vi "MdfCreateDataGroup.vi"(8 "error in (no error)":errorcluster, 10 "ChannelGroupName":string="MDFCGName", 11 "MDFRef":refnum<k24>) -> (0 "error IO":errorcluster, 2 "ChannelGroup":refnum<k24>, 3 "MDFRef out":refnum<k24>)   [LabVIEW 2025, in "MdfFile.lvlib"]
uses:
  MdfFile.lvlib
  data/mdflibrary.dll
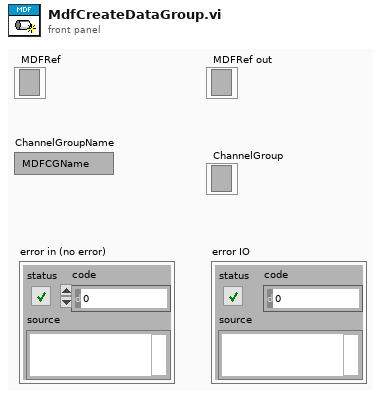
[diagram p1: front panel]
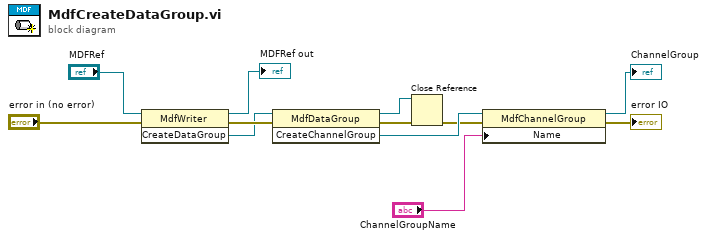
[diagram p0: block diagram]
diagram:
  n1 = invoke class="MdfWriter" method="CreateDataGroup"(reference="MDFRef", error in="error in (no error)") -> (reference out=→"MDFRef out":refnum<k24>, error out=w10:errorcluster, "CreateDataGroup"=w9:refnum<k24>)  [unwired: 1 in]
  n2 = invoke class="MdfDataGroup" method="CreateChannelGroup"(reference=w9, error in=w10) -> (reference out=w7:refnum<k24>, error out=w8:errorcluster, "CreateChannelGroup"=w12:refnum<k24>)  [unwired: 1 in]
  n3 = Close Reference(reference=w7, error in (no error)=w8) -> (error out=w6:errorcluster)
  n4 = property class="MdfChannelGroup"(reference=w12, error in=w6, "Name"="ChannelGroupName") -> (reference out=→"ChannelGroup":refnum<k24>, error out=→"error IO":errorcluster)
